vi "Periodic Tasks.vi"(8 "error in":errorcluster) -> ()   [LabVIEW 2016]
doc: "This VI runs in parallel to other tasks. It can contain as many user-defined periodic loops as you need. These can carry out PID or other sorts of timed response."
uses:
  <vilib>/Rock Robotics/WPI/Utilities/WPI_GetSetVariantRefNum.vi
  Robot Global Data.vi
  <vilib>/Rock Robotics/Network Tables/NT Write Boolean.vi
  <vilib>/Rock Robotics/WPI/RobotDrive/WPI_RobotDriveMecanumDrive_Cartesian.vi
  <vilib>/Rock Robotics/Network Tables/NT Write Numeric Array.vi
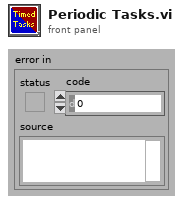
[diagram p1: front panel]
types:
  T1 = typedef "WPI_JoystickDevRef.ctl" = cluster{"Device":T2}
  T2 = typedef "WPI_JoystickDeviceEnum.ctl" = enum16{"USB 0", "USB 1", "USB 2", "USB 3", "USB 4", "USB 5"}
  T3 = typedef "WPI_RobotDriveDevRef.ctl" = cluster{"DevStatus":errorcluster, "Motors[]":T4[], "Square Inputs":bool, "Max Output":dbl}
  T4 = typedef "WPI_MotorControlDeviceRef.ctl" = cluster{"DeviceStatus":errorcluster, "Type":T5, "PWM":cluster{"PWM Channel":T6, "DeadBand":T7}, "CAN":cluster{"Device Number":u8, "SetOutput VI Ref":variant, "GetOutput VI Ref":variant, "Enable VI Ref":variant, "Disable VI Ref":variant, "Data":variant}, "Invert":bool}
  T5 = typedef "WPI_MotorControlType.ctl" = enum16{"PWM", "CAN"}
  T6 = typedef "FPGA_DIOPWMChannel.ctl" = enum8{"PWM 0", "PWM 1", "PWM 2", "PWM 3", "PWM 4", "PWM 5", "PWM 6", "PWM 7", "PWM 8", "PWM 9", "PWM MXP 0", "PWM MXP 1", "PWM MXP 2", "PWM MXP 3", "PWM MXP 4", "PWM MXP 5", "PWM MXP 6", "PWM MXP 7", "PWM MXP 8", "PWM MXP 9", "Invalid"}
  T7 = typedef "WPI_PWMDeadband.ctl" = cluster{"Name":string, "maxPositivePwm":i32, "minPositivePwm":i32, "centerPwm":i32, "maxNegativePwm":i32, "minNegativePwm":i32, "angularRange":u16}
  T8 = cluster{"JoystickDevRef":T1, "RobotDriveDevRef":T3}
  T9 = typedef "WPI_ServoDeviceRef.ctl" = cluster{"DeviceStatus":errorcluster, "PWM Channel":T6, "DeadBand":T7}
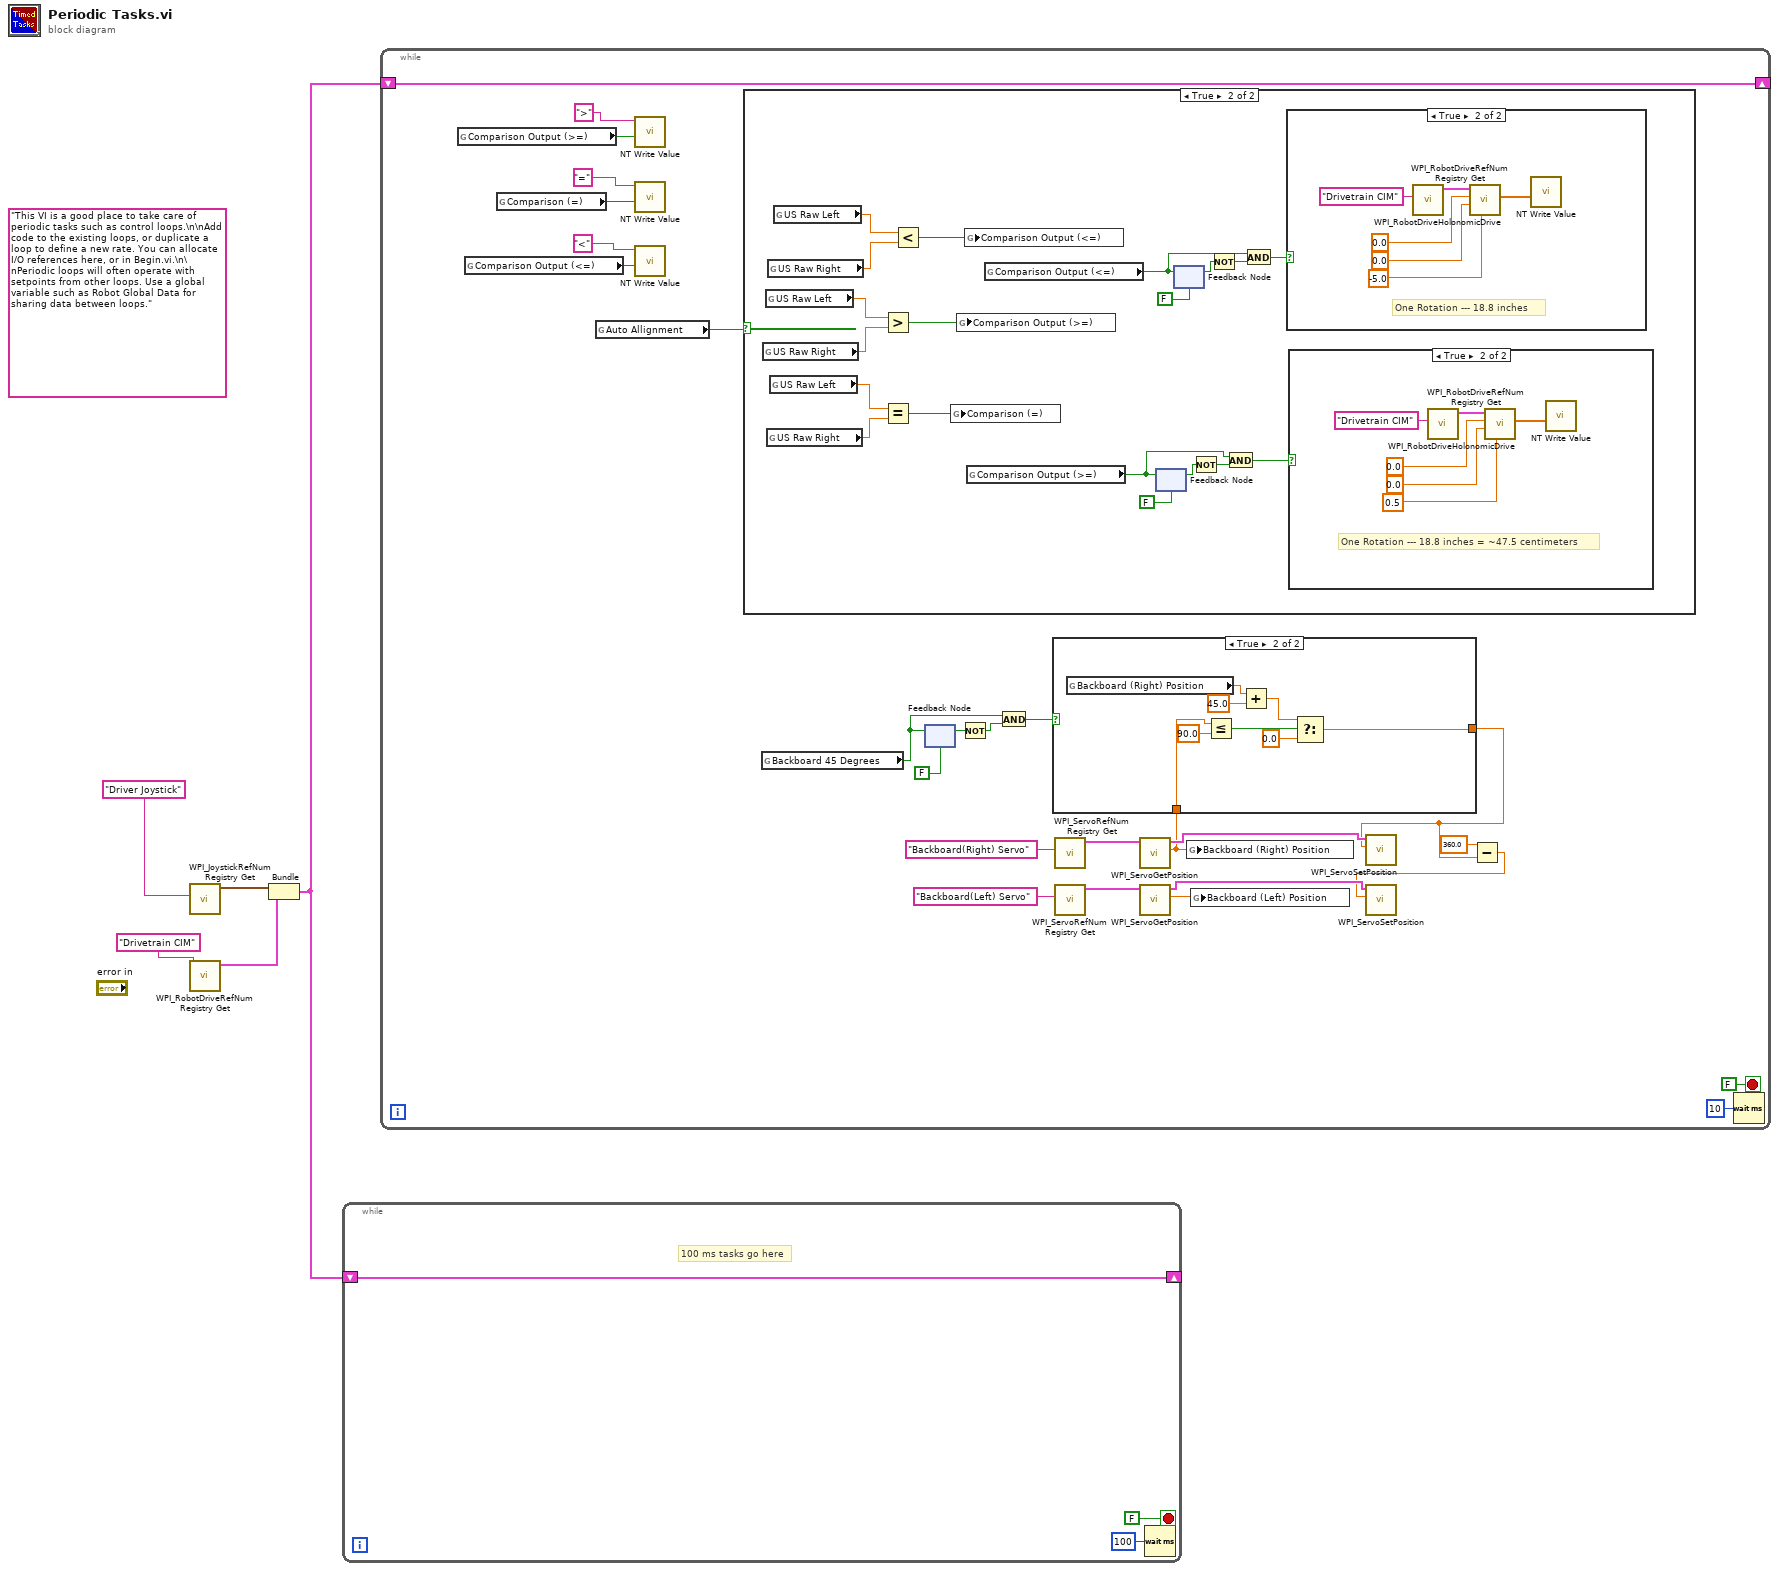
[diagram p0: block diagram]
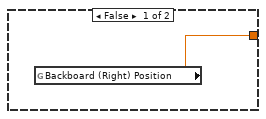
[diagram p2: hidden frame]
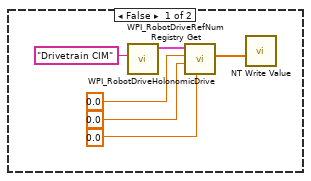
[diagram p4: hidden frame]
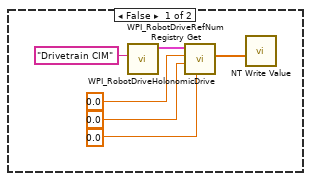
[diagram p5: hidden frame]
diagram:
  (unwired) "This VI is a good place to take care of periodic tasks such as control loops.\n\nAdd code to the existing loops, or duplicate a loop to define a new rate. You can allocate I/O references here, or in Begin.vi.\n\nPeriodic loops will often operate with setpoints from other loops. Use a global variable such as Robot Global Data for sharing data between loops."
  n1 = call <vilib>:"WPI_JoystickRefNum Registry Get.vi"("refnum name"="Driver Joystick") -> ("JoystickDevRef"=w3:T1)  [unwired: 1 in, 9 out]
  n2 = call <vilib>:"WPI_RobotDriveRefNum Registry Get.vi"("refnum name"="Drivetrain CIM") -> ("RobotDriveDevRef"=w2:T3)  [unwired: 1 in, 9 out]
  n3 = Bundle("JoystickDevRef"=w3, "RobotDriveDevRef"=w2) -> (w1:T8)  [unwired: 1 out]
  n4 = while {
    shift-right: [w6] -> _
    shift-left: w1 -> [w6]
    stop <- FALSE stop-if-true
    # "100 ms tasks go here"
    n5 = Wait (ms)(milliseconds to wait=u32 100) -> ()  [unwired: 1 out]
  }
  n6 = while {
    shift-right: [w32] -> _
    shift-left: w1 -> [w32]
    stop <- FALSE stop-if-true
    n7 = global read "Robot Global Data.vi" "Comparison Output (>=)"() -> (w28:bool)
    n8 = global read "Robot Global Data.vi" "Comparison Output (<=)"() -> (w29:bool)
    n9 = global read "Robot Global Data.vi" "Comparison (=)"() -> (w30:bool)
    n10 = global read "Robot Global Data.vi" "Auto Allignment"() -> (w31:bool)
    n11 = call-poly <vilib>:"NT Write Value.vi"("Boolean"=w28, "Name"=">") -> ()  [unwired: 9 in, 1 out]
    n12 = call-poly <vilib>:"NT Write Value.vi"("Boolean"=w30, "Name"="=") -> ()  [unwired: 9 in, 1 out]
    n13 = call-poly <vilib>:"NT Write Value.vi"("Boolean"=w29, "Name"="<") -> ()  [unwired: 9 in, 1 out]
    n14 = case shown="True" w31 {
      frame False {
      }
      frame True {
        n15 = global read "Robot Global Data.vi" "US Raw Right"() -> (w58:dbl)
        n16 = global read "Robot Global Data.vi" "US Raw Left"() -> (w59:dbl)
        n17 = global read "Robot Global Data.vi" "US Raw Right"() -> (w62:dbl)
        n18 = global read "Robot Global Data.vi" "US Raw Right"() -> (w56:dbl)
        n19 = global read "Robot Global Data.vi" "US Raw Left"() -> (w44:dbl)
        n20 = global read "Robot Global Data.vi" "US Raw Left"() -> (w57:dbl)
        n21 = Greater?(x=w59, y=w58) -> (0:w60:bool)
        n22 = Equal?(x=w44, y=w62) -> (x = y?=w61:bool)
        n23 = Less?(x=w57, y=w56) -> (x < y?=w55:bool)
        n24 = global write "Robot Global Data.vi" "Comparison (=)"(w61) -> ()
        n25 = global write "Robot Global Data.vi" "Comparison Output (>=)"(w60) -> ()
        n26 = global write "Robot Global Data.vi" "Comparison Output (<=)"(w55) -> ()
        n27 = global read "Robot Global Data.vi" "Comparison Output (>=)"() -> (w46:bool)
        n28 = global read "Robot Global Data.vi" "Comparison Output (<=)"() -> (w53:bool)
        n29 = feedback #1(FALSE ("Comparison Output (<=)")) -> (w48:bool)
        n30 = feedback-in #1(w46) -> ()
        n31 = feedback-in #2(w53) -> ()
        n32 = feedback #2(FALSE ("Comparison Output (<=)")) -> (w51:bool)
        n33 = Not(x=w48) -> (.not. x?=w47:bool)
        n34 = Not(x=w51) -> (.not. x?=w50:bool)
        n35 = And(x=w46, y=w47) -> (x .and. y?=w45:bool)
        n36 = And(x=w53, y=w50) -> (x .and. y?=w52:bool)
        n37 = case shown="True" w52 {
          frame False {
            n38 = call <vilib>:"WPI_RobotDriveRefNum Registry Get.vi"("refnum name"="Drivetrain CIM") -> ("RobotDriveDevRef"=w80:T3)  [unwired: 9 in, 1 out]
            n39 = call-poly <vilib>:"WPI_RobotDriveHolonomicDrive.vi"("Rotation"=0.0, "Y"=0.0, "X"=0.0, "RobotDriveDevRef"=w80) -> ("Motor Values"=w78:dbl[])  [unwired: 5 in, 2 out]
            n40 = call-poly <vilib>:"NT Write Value.vi"("Numeric Array"=w78) -> ()  [unwired: 10 in, 1 out]
          }
          frame True {
            # "One Rotation --- 18.8 inches"
            n41 = call <vilib>:"WPI_RobotDriveRefNum Registry Get.vi"("refnum name"="Drivetrain CIM") -> ("RobotDriveDevRef"=w86:T3)  [unwired: 9 in, 1 out]
            n42 = call-poly <vilib>:"WPI_RobotDriveHolonomicDrive.vi"("Rotation"=-5.0, "Y"=0.0, "X"=0.0, "RobotDriveDevRef"=w86) -> ("Motor Values"=w84:dbl[])  [unwired: 5 in, 2 out]
            n43 = call-poly <vilib>:"NT Write Value.vi"("Numeric Array"=w84) -> ()  [unwired: 10 in, 1 out]
          }
        }
        n44 = case shown="True" w45 {
          frame False {
            n45 = call <vilib>:"WPI_RobotDriveRefNum Registry Get.vi"("refnum name"="Drivetrain CIM") -> ("RobotDriveDevRef"=w68:T3)  [unwired: 9 in, 1 out]
            n46 = call-poly <vilib>:"WPI_RobotDriveHolonomicDrive.vi"("Rotation"=0.0, "Y"=0.0, "X"=0.0, "RobotDriveDevRef"=w68) -> ("Motor Values"=w66:dbl[])  [unwired: 5 in, 2 out]
            n47 = call-poly <vilib>:"NT Write Value.vi"("Numeric Array"=w66) -> ()  [unwired: 10 in, 1 out]
          }
          frame True {
            # "One Rotation --- 18.8 inches = ~47.5 centimeters"
            n48 = call <vilib>:"WPI_RobotDriveRefNum Registry Get.vi"("refnum name"="Drivetrain CIM") -> ("RobotDriveDevRef"=w74:T3)  [unwired: 9 in, 1 out]
            n49 = call-poly <vilib>:"WPI_RobotDriveHolonomicDrive.vi"("Rotation"=0.5, "Y"=0.0, "X"=0.0, "RobotDriveDevRef"=w74) -> ("Motor Values"=w72:dbl[])  [unwired: 5 in, 2 out]
            n50 = call-poly <vilib>:"NT Write Value.vi"("Numeric Array"=w72) -> ()  [unwired: 10 in, 1 out]
          }
        }
      }
    }
    n51 = global read "Robot Global Data.vi" "Backboard 45 Degrees"() -> (w19:bool)
    n52 = feedback #3(FALSE) -> (w21:bool)
    n53 = feedback-in #3(w19) -> ()
    n54 = Not(x=w21) -> (.not. x?=w13:bool)
    n55 = And(x=w19, y=w13) -> (x .and. y?=w20:bool)
    n56 = call <vilib>:"WPI_ServoRefNum Registry Get.vi"("refnum name"="Backboard(Right) Servo") -> ("ServoDeviceRef"=w24:T9)  [unwired: 9 in, 1 out]
    n57 = call <vilib>:"WPI_ServoRefNum Registry Get.vi"("refnum name"="Backboard(Left) Servo") -> ("ServoDeviceRef"=w17:T9)  [unwired: 9 in, 1 out]
    n58 = call <vilib>:"WPI_ServoGetPosition.vi"("ServoDeviceRef"=w24) -> ("Position"=w9:dbl, "ServoDeviceRef"=w23:T9)  [unwired: 8 in, 1 out]
    n59 = case shown="True" w20 {
      tunnel: [w35 w40] -> w11
      tunnel: w9 -> [_ w36]
      frame False {
        n60 = global read "Robot Global Data.vi" "Backboard (Right) Position"() -> (w35:dbl)
      }
      frame True {
        n61 = global read "Robot Global Data.vi" "Backboard (Right) Position"() -> (w39:dbl)
        n62 = Less Or Equal?(x=w36, y=90.0) -> (x <= y?=w38:bool)
        n63 = Add(x=w39, y=45.0) -> (x+y=w43:dbl)
        n64 = Select(t=w43, s=w38, f=0.0) -> (s? t:f=w40:dbl)
      }
    }
    n65 = call <vilib>:"WPI_ServoGetPosition.vi"("ServoDeviceRef"=w17) -> ("Position"=w15:dbl, "ServoDeviceRef"=w16:T9)  [unwired: 8 in, 1 out]
    n66 = global write "Robot Global Data.vi" "Backboard (Right) Position"(w9) -> ()
    n67 = global write "Robot Global Data.vi" "Backboard (Left) Position"(w15) -> ()
    n68 = call <vilib>:"WPI_ServoSetPosition.vi"("Position"=w11, "ServoDeviceRef"=w23) -> ()  [unwired: 8 in, 2 out]
    n69 = Subtract(x=360.0, y=w11) -> (x-y=w10:dbl)
    n70 = call <vilib>:"WPI_ServoSetPosition.vi"("Position"=w10, "ServoDeviceRef"=w16) -> ()  [unwired: 8 in, 2 out]
    n71 = Wait (ms)(milliseconds to wait=u32 10) -> ()  [unwired: 1 out]
  }
